vi "Read Listening Queue.vi"(8 "error in (no error)":errorcluster, 11 "Generic Controller in":refnum<class "Generic Plugin.lvclass">) -> (0 "error out":errorcluster, 2 "Listening Queue":refnum<queue>, 3 "Generic Controller out":refnum<class "Generic Plugin.lvclass">)   [LabVIEW 2020, in "Generic Plugin.lvclass"]
uses:
  Generic Plugin.lvclass
  <userlib>/Dynamic Reentrant/Type Defs/Message.ctl
  <userlib>/Dynamic Reentrant/Dynamic Reentrant.lvlib
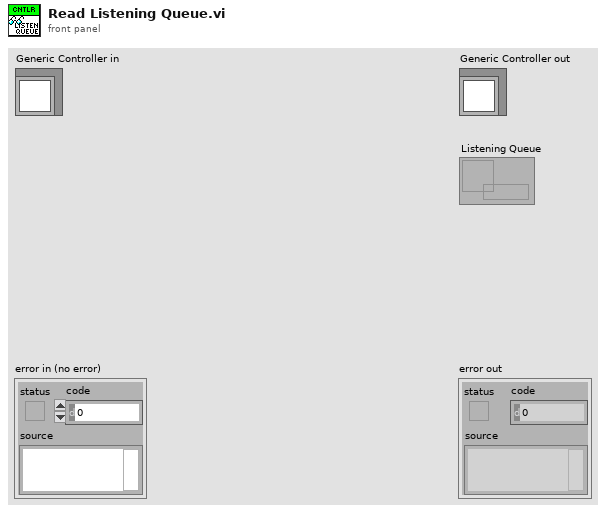
[diagram p1: front panel]
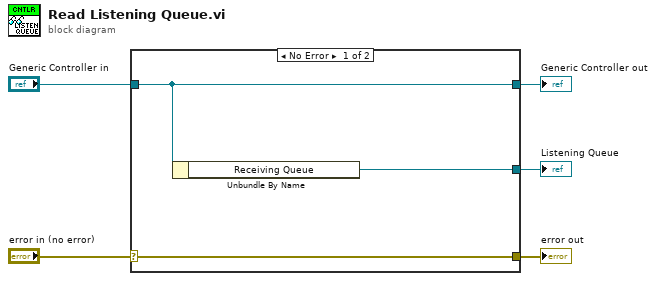
[diagram p0: block diagram]
diagram:
  n1 = case shown="No Error" "error in (no error)" {
    selector: "error in (no error)" -> [w8 w9]
    tunnel: [w8 w9] -> w4
    tunnel: [w7 w10] -> w2
    tunnel: "Generic Controller in" -> [w7 w10]
    tunnel: [w6 _] -> w1
    frame No Error {
      n2 = Unbundle By Name(w7) -> ("Receiving Queue"=w6:refnum<queue>)
    }
    frame Error {
    }
  }
  "error out" <- w4
  "Generic Controller out" <- w2
  "Listening Queue" <- w1
